vi "Get Status.vi"(8 "error in (no error)":errorcluster, 11 "Sync Box in":refnum<class "Sync Box.lvclass">) -> (0 "error out":errorcluster, 2 "data out":string, 3 "Sync Box out":refnum<class "Sync Box.lvclass">)   [LabVIEW 2012, in "Sync Box.lvclass"]
uses:
  Sync Box.lvclass
  Sync Box.lvclass/Sync Box.ctl
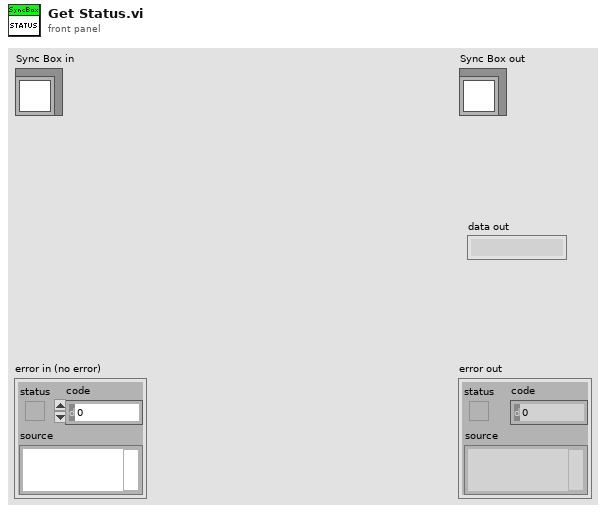
[diagram p1: front panel]
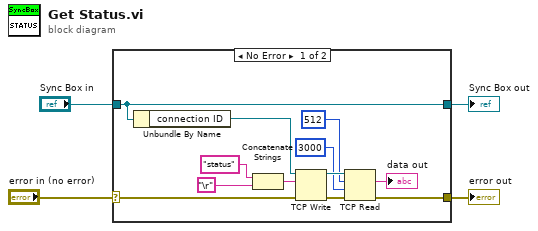
[diagram p0: block diagram]
diagram:
  n1 = case shown="No Error" "error in (no error)" {
    selector: "error in (no error)" -> [w14 w18]
    tunnel: [w5 w18] -> w2
    tunnel: "Sync Box in" -> [w11 w17]
    tunnel: [w11 w17] -> w1
    frame No Error {
      n2 = Unbundle By Name(w11) -> ("connection ID"=w12:refnum<k5>)
      n3 = Concatenate Strings("status", "\r") -> (w16:string)
      n4 = TCP Write(connection ID=w12, data in=w16, error in (no error)=w14) -> (connection ID out=w10:refnum<k5>, error out=w9:errorcluster)  [unwired: 1 in, 1 out]
      n5 = TCP Read(connection ID=w10, bytes to read=512, error in (no error)=w9, 9:3000 ("timeout ms (25000)")) -> (data out=→"data out":string, error out=w5:errorcluster)  [unwired: 1 in, 1 out]
    }
    frame Error {
    }
  }
  "error out" <- w2
  "Sync Box out" <- w1
